vi "FeedbackDecode_BarPlotKinematics.vi"() -> ()   [LabVIEW 2020]
uses:
  <vilib>/Utility/miscctls.llb/LVBoundsTypeDef.ctl
  FeedbackDecode_Globals.vi
panel:
  in  "[user-specified font]":T1={"Font Name:"="Arial", "Size"=36, "Strikeout?"=FALSE, "Italic?"=FALSE, "Underline?"=FALSE, "Outline?"=FALSE, "Shadow?"=FALSE, "Bold?"=TRUE}
  out "Draw Area Size":T2={"Width"=762, "Height"=186}
  in  "KinLabels":string[](array[string])=["Thumb", "Index", "Middle", "Ring", "Pinky", "ThumbInt", "IndexInt", "RingInt", "LittleInt", "WristPitch", "WristYaw", "WristRoll"]
  out "Pic":picture
  out "Bar":cluster{i32, dbl}[](graph)
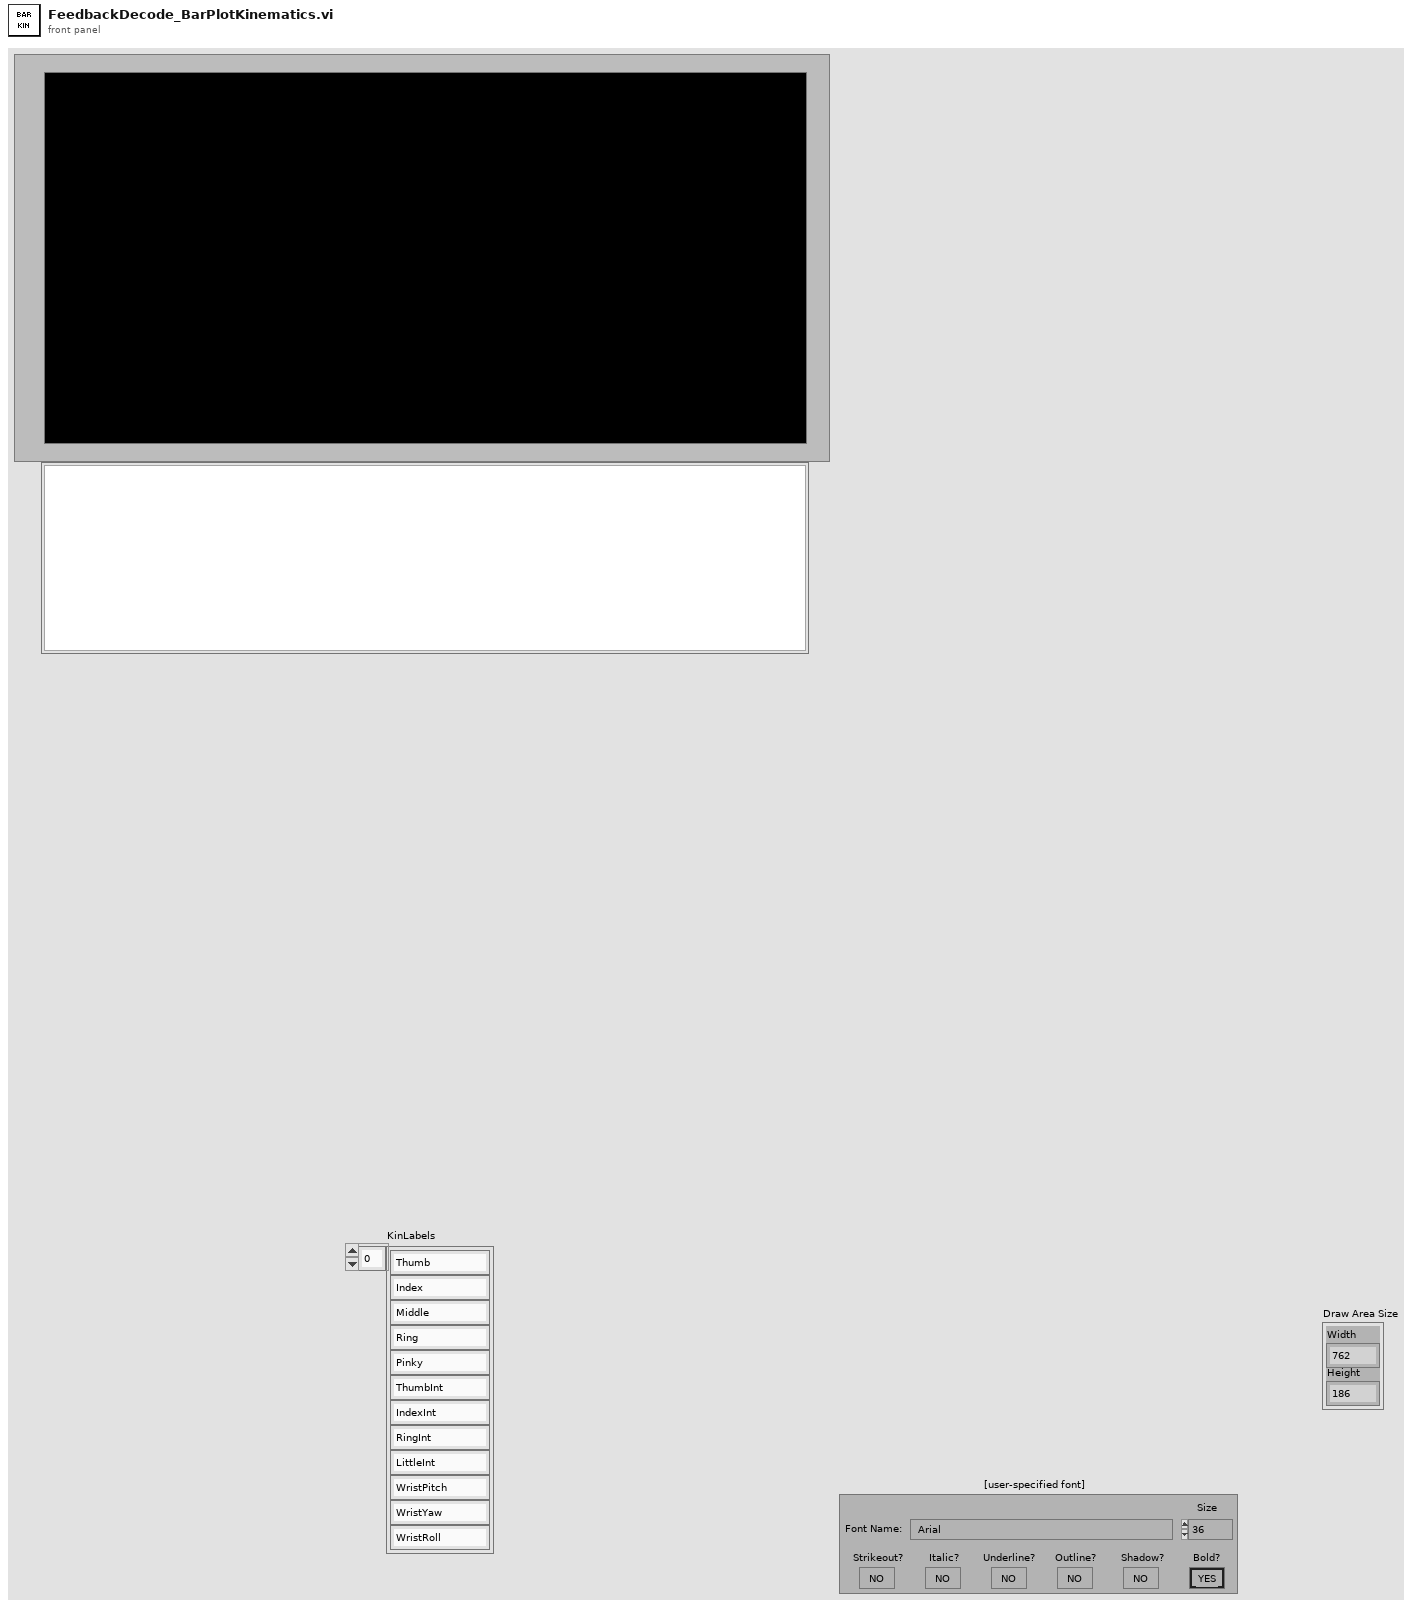
[diagram p1: front panel]
types:
  T1 = cluster{"Font Name:":string, "Size":i16, "Strikeout?":bool, "Italic?":bool, "Underline?":bool, "Outline?":bool, "Shadow?":bool, "Bold?":bool}
  T2 = typedef "LVBoundsTypeDef.ctl" = cluster{"Width":u32, "Height":u32}
  T3 = enum16{"User-specified Font", "Application Font", "System Font", "Dialog Font"}
  T4 = enum16{"None", "Stacked", "Clockwise", "Counterclockwise"}
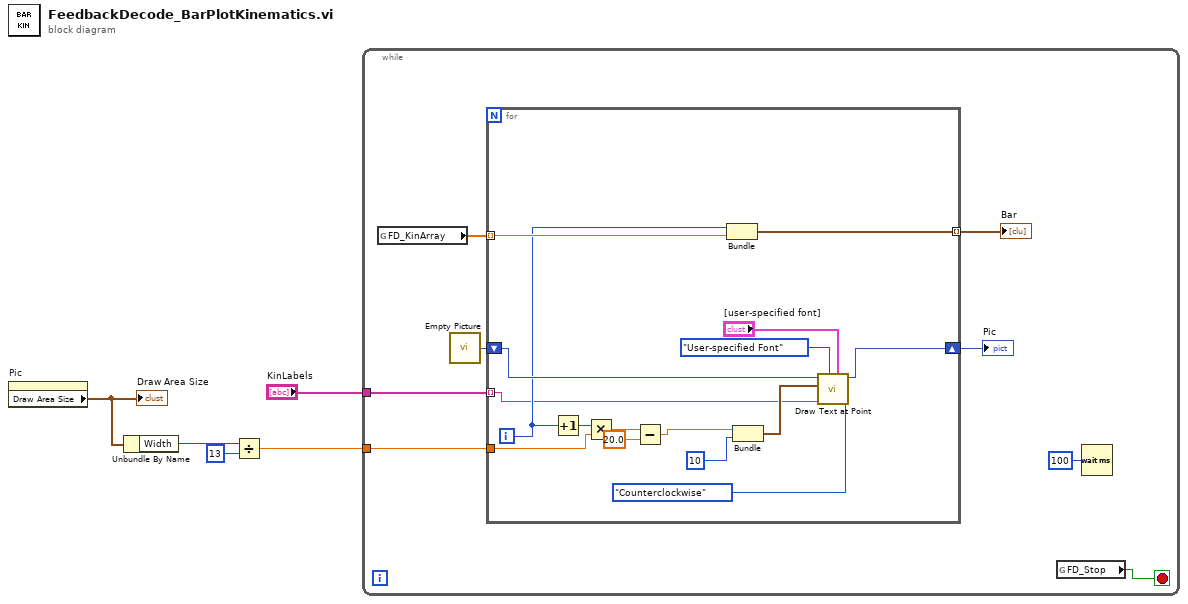
[diagram p0: block diagram]
diagram:
  n1 = property on="Pic" class="Pict"() -> ("Draw Area Size"=w1:T2)  [unwired: 2 in, 2 out]
  "Draw Area Size" <- w1
  n2 = Unbundle By Name(w1) -> ("Width"=w4:u32)
  n3 = Divide(x=w4, y=u32 13) -> (x/y=w2:dbl)
  n4 = while {
    tunnel: "KinLabels" -> [w12]
    tunnel: w2 -> [w9]
    stop <- w8 stop-if-true
    n5 = global read "FeedbackDecode_Globals.vi" "FD_KinArray"() -> (w6:dbl[])
    n6 = call "Empty Picture"() -> ("empty picture"=w11:picture)
    n7 = for {
      tunnel: w6 -> [w28] mode=indexing
      tunnel: [w29] -> w13 mode=indexing
      tunnel: w12 -> [w20] mode=indexing
      shift-right: [w26] -> w10
      shift-left: w11 -> [w27]
      tunnel: w9 -> [w17]
      i -> [w25]
      n8 = Increment(x=w25) -> (x+1=w24:i32)
      n9 = Multiply(x=w24, y=w17) -> (x*y=w16:dbl)
      n10 = Subtract(x=w16, y=20.0) -> (x-y=w15:dbl)
      n11 = Bundle(w25, "Thumb"=w28) -> (w29:cluster{i32, "Thumb":dbl})  [unwired: 1 in]
      n12 = Bundle(w15, "y"=10) -> (w21:cluster{dbl, "y":i32})  [unwired: 1 in]
      n13 = call <vilib>:"Draw Text at Point.vi"("text orientation"=T4."Counterclockwise", "[user-specified font]"="[user-specified font]", "desired font(Application)"=T3."User-specified Font", "text"=w20, "origin"=w21, "picture"=w27) -> ("new picture"=w26:picture)  [unwired: 4 in, 1 out]
    }
    "Bar" <- w13
    "Pic" <- w10
    n14 = global read "FeedbackDecode_Globals.vi" "FD_Stop"() -> (w8:bool)
    n15 = Wait (ms)(milliseconds to wait=u32 100) -> ()  [unwired: 1 out]
  }
